vi "Send Message.vi"(8 "Error In":errorcluster, 10 "IMessage":refnum<class "IMessage.lvclass">, 11 "Communicator in":refnum<class "Communicator.lvclass">) -> (0 "Error Out":errorcluster, 3 "Communicator out":refnum<class "Communicator.lvclass">)   [LabVIEW 2024, in "Communicator.lvclass"]
uses:
  Communicator.lvclass
  Source/Interfaces/IMessage/IMessage.lvclass
  Source/Interfaces/ICommunicate/ICommunicate.lvclass
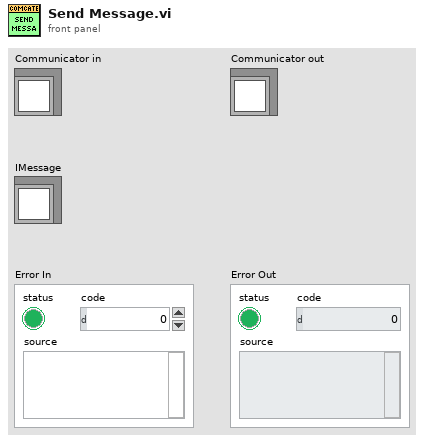
[diagram p1: front panel]
types:
  T1 = typedef "Communicator.lvclass/ObjectAttributes.ctl" = cluster{"IConfigure":refnum<class "IConfigure.lvclass">}
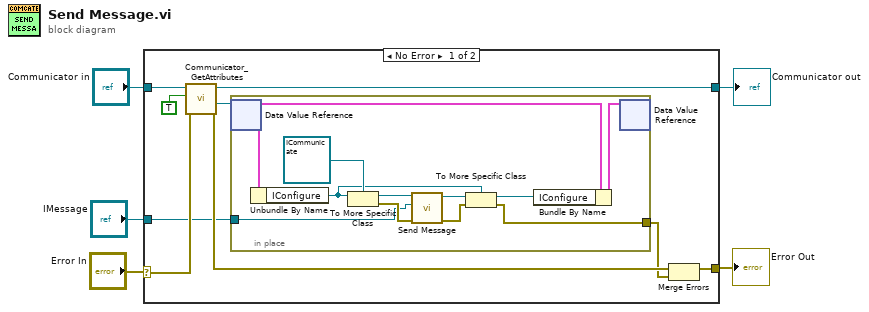
[diagram p0: block diagram]
diagram:
  n1 = case shown="No Error" "Error In" {
    selector: "Error In" -> [w13 w27]
    tunnel: [w11 w27] -> w4
    tunnel: [w12 w26] -> w2
    tunnel: "Communicator in" -> [w14 w26]
    tunnel: "IMessage" -> [w7 _]
    frame No Error {
      n2 = call "Communicator_GetAttributes.vi"("Error In"=w13, "OnlyGetDvrReference(False)"=TRUE, "Communicator in"=w14) -> ("Error Out"=w9:errorcluster, "DataRef"=w10:refnum<data-value>, "Communicator out"=w12:refnum<class "Communicator.lvclass">)  [unwired: 5 in, 1 out]
      n3 = in-place {
        in-place-border: w7 -> [w15]
        in-place-border: [w16] -> w6
        n4 = in-place-dvr #1(w10) -> (w24:T1)  [unwired: 1 out]
        n5 = Unbundle By Name(w24) -> ("IConfigure"=w18:refnum<class "IConfigure.lvclass">)
        n6 = To More Specific Class(target class=refnum<class "ICommunicate.lvclass"> refnum ("ICommunicate.lvclass"), reference=w18) -> (specific class reference=w21:refnum<class "ICommunicate.lvclass">, error out=w22:errorcluster)  [unwired: 1 in]
        n7 = call-dynamic "Send Message.vi"("error in"=w22, "IMessage"=w15, "ICommunicate in"=w21) -> ("error out"=w17:errorcluster, "ICommunicate out"=w20:refnum<class "ICommunicate.lvclass">)  [unwired: 7 in]
        n8 = To More Specific Class(target class=w18, reference=w20, error in=w17) -> (specific class reference=w19:refnum<class "IConfigure.lvclass">, error out=w16:errorcluster)
        n9 = Bundle By Name(cluster=w24, "IConfigure"=w19) -> (w25:T1)
        n10 = in-place-dvr #1(w25) -> ()  [unwired: 2 out]
      }
      n11 = Merge Errors(w9, w6) -> (w11:errorcluster)
    }
    frame Error {
    }
  }
  "Error Out" <- w4
  "Communicator out" <- w2
